vi "convert(SubVI).vi"(11 "String in":string) -> (2 "Errors":dbl[][](array[numeric]), 3 "PIDs":dbl[](array[numeric]))   [LabVIEW 2017]
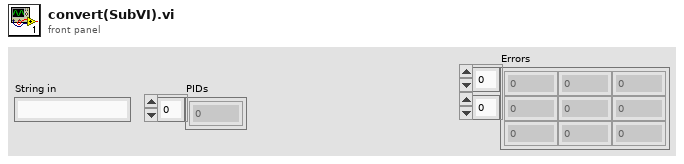
[diagram p1: front panel]
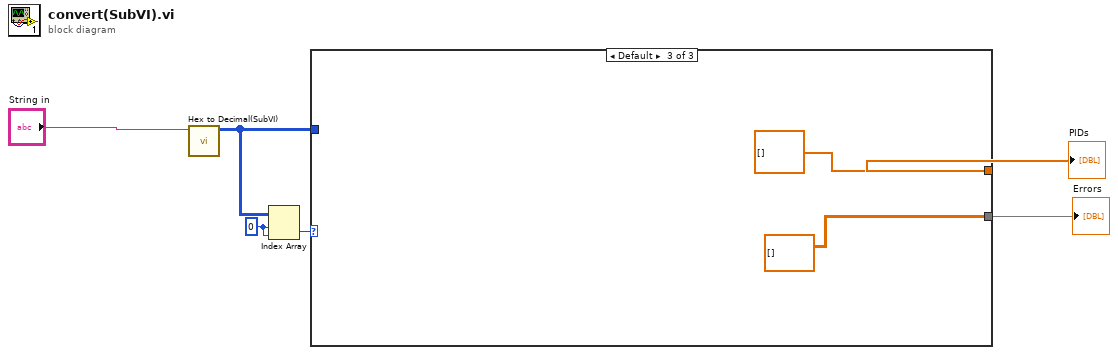
[diagram p0: block diagram]
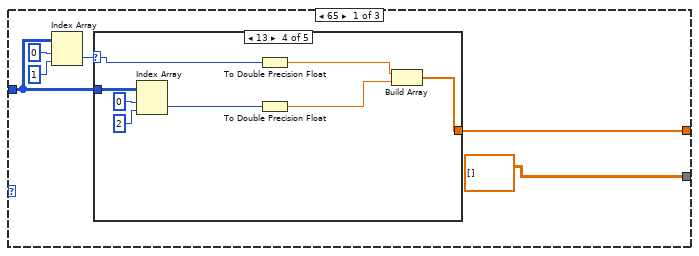
[diagram p2: hidden frame]
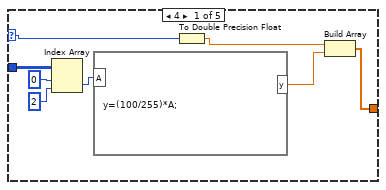
[diagram p3: hidden frame]
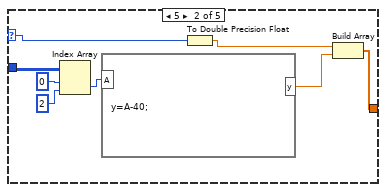
[diagram p4: hidden frame]
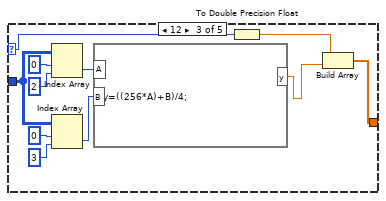
[diagram p5: hidden frame]
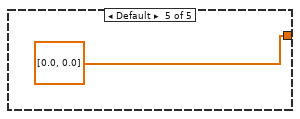
[diagram p6: hidden frame]
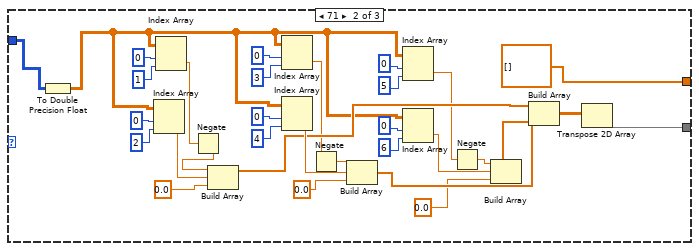
[diagram p7: hidden frame]
diagram:
  w4 = 0 ("index (row)")
  n1 = call "Hex to Decimal(SubVI).vi"("String in"="String in") -> ("Array"=w2:u32[][])  [unwired: 10 in]
  n2 = Index Array(array=w2, index (row)=w4, index (col)=w4) -> (element=w5:u32)
  n3 = case shown="Default" w5 {
    tunnel: w2 -> [w9 w58 _]
    tunnel: [w8 dbl[] [] dbl[] []] -> w6
    tunnel: [dbl[][] [] w59 dbl[][] []] -> w1
    frame 65 {
      n4 = Index Array(array=w9, index (row)=0, index (col)=1 ("index (row)")) -> (element=w10:u32)
      n5 = case shown="13" w10 {
        selector: w10 -> [w16 w22 w32 w43 _]
        tunnel: w9 -> [w18 w23 w36 w45 _]
        tunnel: [w15 w21 w29 w40 dbl[] [0.0, 0.0]] -> w8
        frame 4 {
          n6 = Index Array(array=w18, index (row)=0 ("disabled index (col)"), index (col)=2 ("disabled index (col)")) -> (element=w17:u32)
          n7 = formula code="y=(100/255)*A;"("A"=w17) -> ("y"=w13:dbl)
          n8 = To Double Precision Float(number=w16) -> (double precision float=w14:dbl)
          n9 = Build Array(w14, w13) -> (w15:dbl[])
        }
        frame 5 {
          n10 = Index Array(array=w23, index (row)=0 ("disabled index (col)"), index (col)=2 ("disabled index (col)")) -> (element=w26:u32)
          n11 = formula code="y=A-40;"("A"=w26) -> ("y"=w24:dbl)
          n12 = To Double Precision Float(number=w22) -> (double precision float=w25:dbl)
          n13 = Build Array(w25, w24) -> (w21:dbl[])
        }
        frame 12 {
          n14 = Index Array(array=w36, index (row)=0 ("disabled index (col)"), index (col)=2 ("disabled index (col)")) -> (element=w35:u32)
          n15 = Index Array(array=w36, index (row)=0 ("disabled index (col)"), index (col)=3 ("disabled index (col)")) -> (element=w34:u32)
          n16 = formula code="y=((256*A)+B)/4;"("A"=w35, "B"=w34) -> ("y"=w30:dbl)
          n17 = To Double Precision Float(number=w32) -> (double precision float=w31:dbl)
          n18 = Build Array(w31, w30) -> (w29:dbl[])
        }
        frame 13 {
          n19 = Index Array(array=w45, index (row)=0 ("disabled index (col)"), index (col)=2 ("disabled index (col)")) -> (element=w44:u32)
          n20 = To Double Precision Float(number=w43) -> (double precision float=w42:dbl)
          n21 = To Double Precision Float(number=w44) -> (double precision float=w41:dbl)
          n22 = Build Array(w42, w41) -> (w40:dbl[])
        }
        frame Default {
        }
      }
    }
    frame 71 {
      n23 = To Double Precision Float(number=w58) -> (double precision float=w57:dbl[][])
      n24 = Index Array(array=w57, index (row)=0, index (col)=2 ("index (row)")) -> (element=w73:dbl)
      n25 = Index Array(array=w57, index (row)=0, index (col)=1 ("index (row)")) -> (element=w56:dbl)
      n26 = Negate(x=w56) -> (-x=w55:dbl)
      n27 = Build Array(w55, w73, 0.0 ("element")) -> (w64:dbl[])
      n28 = Index Array(array=w57, index (row)=0, index (col)=3 ("index (row)")) -> (element=w51:dbl)
      n29 = Index Array(array=w57, index (row)=0, index (col)=4 ("index (row)")) -> (element=w72:dbl)
      n30 = Negate(x=w51) -> (-x=w52:dbl)
      n31 = Build Array(w52, w72, 0.0 ("element")) -> (w63:dbl[])
      n32 = Index Array(array=w57, index (row)=0, index (col)=5 ("index (row)")) -> (element=w49:dbl)
      n33 = Index Array(array=w57, index (row)=0, index (col)=6 ("index (row)")) -> (element=w65:dbl)
      n34 = Negate(x=w49) -> (-x=w50:dbl)
      n35 = Build Array(w50, w65, 0.0 ("element")) -> (w62:dbl[])
      n36 = Build Array(w64, w63, w62) -> (w61:dbl[][])
      n37 = Transpose 2D Array(2D array=w61) -> (transposed array=w59:dbl[][])
    }
    frame Default {
    }
  }
  "PIDs" <- w6
  "Errors" <- w1
